vi "Check for error chatting.vi"(8 "error in (no error)":errorcluster, 11 "VISA resource name":refnum<visa-resource-name>) -> (0 "error out":errorcluster, 2 "Error chatting?":bool, 3 "VISA resource name out":refnum<visa-resource-name>)   [LabVIEW 2013]
panel:
  out "read buffer":string
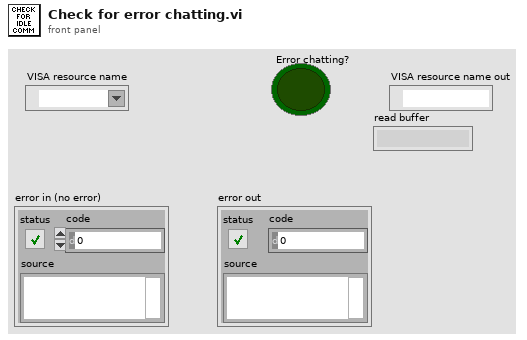
[diagram p1: front panel]
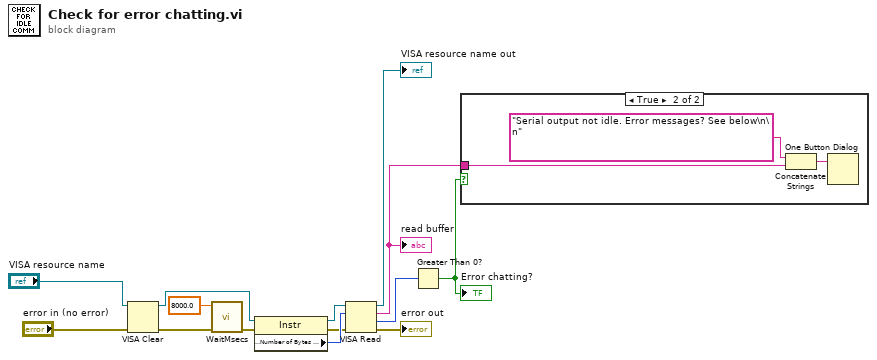
[diagram p0: block diagram]
diagram:
  n1 = VISA Clear(VISA resource name="VISA resource name", error in (no error)="error in (no error)") -> (VISA resource name out=w9:refnum<visa-resource-name>, error out=w12:errorcluster)
  n2 = call "WaitMsecs.vi"("error in (no error)"=w12, "Wait Msecs"=8000.0) -> ("error out"=w10:errorcluster)  [unwired: 9 in]
  n3 = property class="Instr"(reference=w9, error in=w10) -> (reference out=w6:refnum<visa-resource-name>, error out=w7:errorcluster, "Serial Settings:Number of Bytes at Serial Port"=w8:u32)
  n4 = VISA Read(VISA resource name=w6, byte count=w8, error in (no error)=w7) -> (VISA resource name out=→"VISA resource name out":refnum<visa-resource-name>, read buffer=w1:string, return count=w5:u32, error out=→"error out":errorcluster)
  "read buffer" <- w1
  n5 = Greater Than 0?(x=w5) -> (x > 0?=w2:bool)
  "Error chatting?" <- w2
  n6 = case shown="True" w2 {
    tunnel: w1 -> [_ w16]
    frame False {
    }
    frame True {
      n7 = Concatenate Strings("Serial output not idle. Error messages? See below\n\n" ("string"), w16) -> (w15:string)
      n8 = One Button Dialog(message=w15) -> ()  [unwired: 1 in, 1 out]
    }
  }
